vi "PicoScope6000GetRapidBlock.vi"(0 "error in":errorcluster, 7 "handle in":i16, 11 "Rapid Block Acquisition Settings":T1) -> (2 "Channel A Buffer":i16[][](array[numeric]), 3 "Channel B Buffer":i16[][](array[numeric]), 4 "error out":errorcluster, 6 "handle out":i16, 13 "Channel C Buffer":i16[][](array[numeric]), 14 "Channel D Buffer":i16[][](array[numeric]))   [LabVIEW 2009]
doc: "This VI gets a set of blocks captured using rapid block mode. It outputs two-dimensional arrays for each channel that contain data from all the requested captures."
uses:
  PS6000.dll
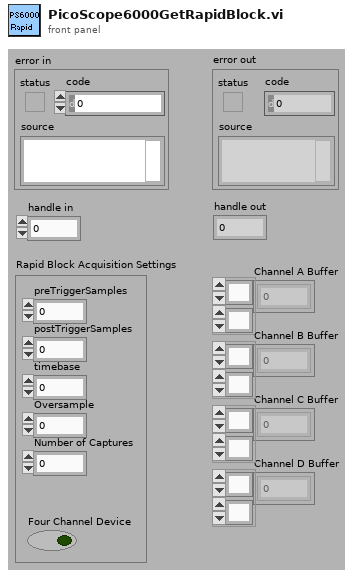
[diagram p1: front panel]
types:
  T1 = cluster{"preTriggerSamples":u32, "postTriggerSamples":u32, "timebase":u32, "Four Channel Device":bool, "Oversample":i16, "Number of Captures":u32}
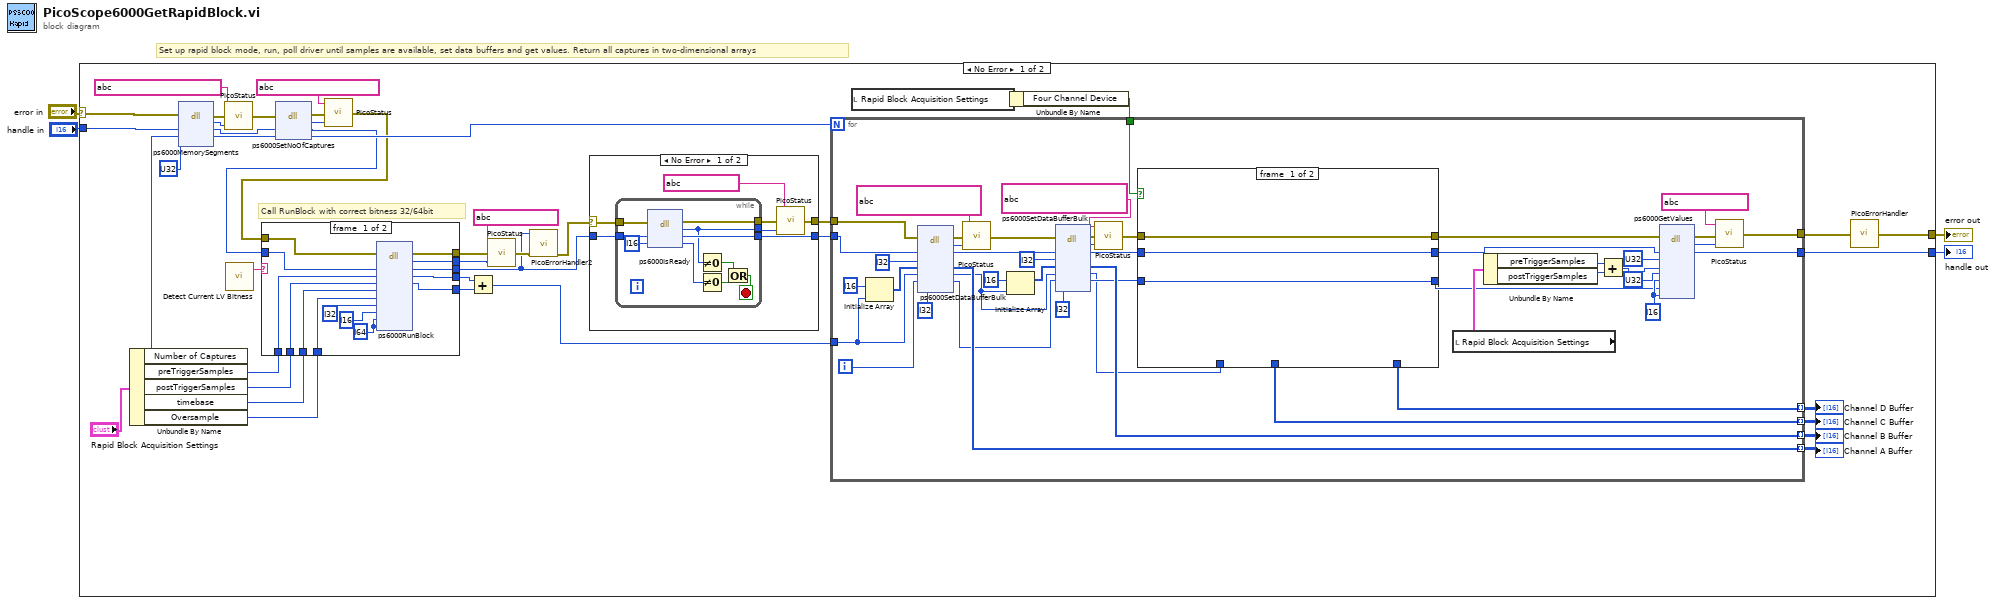
[diagram p0: block diagram]
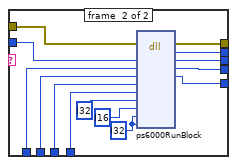
[diagram p2: hidden frame]
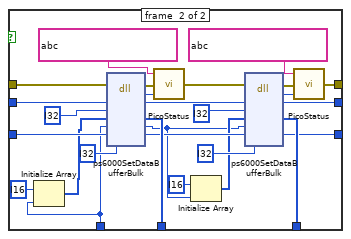
[diagram p3: hidden frame]
diagram:
  # "Set up rapid block mode, run, poll driver until samples are available, set data buffers and get values. Return all captures in two-dimensional arrays"
  n1 = case shown="No Error" "error in" {
    selector: "error in" -> [w42 w171]
    tunnel: [w21 w171] -> w3
    tunnel: "handle in" -> [w41 w170]
    tunnel: [w23 w170] -> w1
    frame #0 {
      # "Call RunBlock with correct bitness 32/64bit"
      n2 = Unbundle By Name("Rapid Block Acquisition Settings") -> ("Number of Captures"=w37:u32, "preTriggerSamples"=w9:u32, "postTriggerSamples"=w8:u32, "timebase"=w7:u32, "Oversample"=w6:i16)
      n3 = dll-call lib="PS6000.dll" fn="ps6000MemorySegments" ("ps3000.dll:_ps3000_open_unit@0")(error in=w42, "handle"=w41, "nSegments"=w37, "nMaxSamples"=u32 ?) -> (error out=w39:errorcluster, "PICO_STATUS"=w40:i32, "handle"=w34:i16, "nSegments"=w35:u32)  [unwired: 3 in, 1 out]
      n4 = call "PicoStatus.vi"("PICO STATUS"=w40, "error in"=w39, "source"=string ?) -> ("error out"=w33:errorcluster)
      n5 = call "Detect Current LV Bitness.vi"() -> ("bitness"=w16:string)  [unwired: 11 in]
      n6 = dll-call lib="PS6000.dll" fn="ps6000SetNoOfCaptures" ("ps3000.dll:_ps3000_open_unit@0")(error in=w33, "handle"=w34, "nCaptures"=w35) -> (error out=w31:errorcluster, "PICO_STATUS"=w32:i32, "handle"=w12:i16, "nCaptures"=w28:u32)  [unwired: 2 in, 1 out]
      n7 = call "PicoStatus.vi"("PICO STATUS"=w32, "error in"=w31, "source"=string ?) -> ("error out"=w13:errorcluster)
      n8 = case shown="\"32\", Default" w16 {
        tunnel: w7 -> [w60 w74]
        tunnel: w9 -> [w59 w73]
        tunnel: w8 -> [w58 w72]
        tunnel: [w57 w71] -> w20
        tunnel: [w56 w70] -> w19
        tunnel: w13 -> [w55 w69]
        tunnel: w12 -> [w54 w68]
        tunnel: w6 -> [w53 w67]
        tunnel: [w52 w66] -> w10
        tunnel: [w48 w62] -> w15
        tunnel: [w47 w61] -> w14
        frame #0 {
          w50 = i64 ? ("pParameter")
          n9 = dll-call lib="PS6000.dll" fn="ps6000RunBlock" ("ps3000.dll:_ps3000_open_unit@0")(error in=w55, "handle"=w54, "preTriggerSamples"=w59, "postTriggerSamples"=w58, "timebase"=w60, "oversample"=w53, "timeindisposed"=i32 ? ("pParameter"), "segmentIndex"=i16 ? ("pParameter"), "lpReady"=w50, "pParameter"=w50) -> (error out=w56:errorcluster, "PICO_STATUS"=w57:u32, "handle"=w52:i16, "preTriggerSamples"=w47:u32, "postTriggerSamples"=w48:u32)  [unwired: 8 in, 1 out]
        }
        frame #1 {
          w64 = i32 ? ("pParameter")
          n10 = dll-call lib="PS6000.dll" fn="ps6000RunBlock" ("ps3000.dll:_ps3000_open_unit@0")(error in=w69, "handle"=w68, "preTriggerSamples"=w73, "postTriggerSamples"=w72, "timebase"=w74, "oversample"=w67, "timeindisposed"=i32 ? ("pParameter"), "segmentIndex"=i16 ? ("pParameter"), "lpReady"=w64, "pParameter"=w64) -> (error out=w70:errorcluster, "PICO_STATUS"=w71:u32, "handle"=w66:i16, "preTriggerSamples"=w61:u32, "postTriggerSamples"=w62:u32)  [unwired: 8 in, 1 out]
        }
      }
      n11 = Add(x=w14, y=w15) -> (x+y=w5:u32)
      n12 = call "PicoStatus.vi"("PICO STATUS"=w20, "error in"=w19, "source"=string ?) -> ("error out"=w17:errorcluster)
      n13 = call "PicoErrorHandler2.vi"("error in (no error)"=w17, "handle In"=w10) -> ("error out"=w11:errorcluster)  [unwired: 9 in]
      n14 = case shown="No Error" w11 {
        selector: w11 -> [w155 w168]
        tunnel: w10 -> [w157 w169]
        tunnel: [w156 w169] -> w46
        tunnel: [w154 w168] -> w45
        frame #0 {
          n15 = while {
            tunnel: [w167] -> w156
            tunnel: w157 -> [w166]
            tunnel: [w161] -> w152
            tunnel: w155 -> [w160]
            tunnel: [w159] -> w153
            stop <- w165 stop-if-true
            n16 = dll-call lib="PS6000.dll" fn="ps6000IsReady" ("ps3000.dll:_ps3000_open_unit@0")(error in=w160, "handle"=w166, "ready"=i16 ?) -> (error out=w159:errorcluster, "status"=w161:i32, "handle"=w167:i16, "ready"=w162:i16)  [unwired: 2 in, 1 out]
            n17 = Not Equal To 0?(x=w161) -> (x != 0?=w163:bool)
            n18 = Not Equal To 0?(x=w162) -> (x != 0?=w164:bool)
            n19 = Or(x=w163, y=w164) -> (x .or. y?=w165:bool)
          }
          n20 = call "PicoStatus.vi"("PICO STATUS"=w152, "error in"=w153, "source"=string ?) -> ("error out"=w154:errorcluster)
        }
        frame #1 {
        }
      }
      n21 = local read "Rapid Block Acquisition Settings"() -> (w29:T1)
      n22 = Unbundle By Name(w29) -> ("Four Channel Device"=w43:bool)
      n23 = for {
        N: w28 -> [_]
        tunnel: w46 -> [w120]
        tunnel: w45 -> [w115]
        tunnel: w43 -> [w106]
        tunnel: [w109] -> w27 mode=indexing
        tunnel: [w108] -> w26 mode=indexing
        tunnel: [w82] -> w25 mode=indexing
        tunnel: [w104] -> w24 mode=indexing
        tunnel: w5 -> [w107]
        tunnel: [w91] -> w23
        tunnel: [w77] -> w22
        i -> [w105]
        w103 = i16 ? ("overflow")
        n24 = Initialize Array(i16 ? ("element"), w107) -> (w119:i16[])
        n25 = dll-call lib="PS6000.dll" fn="ps6000SetDataBufferBulk" ("ps3000.dll:_ps3000_open_unit@0")(error in=w115, "handle"=w120, "channel"=i32 ?, "buffer"=w119, "bufferLth"=w107, "waveform"=w105, "downSampleRatioMode"=i32 ?) -> (error out=w113:errorcluster, "PICO_STATUS"=w114:i32, "handle"=w87:i16, "buffer"=w104:i16[], "bufferLth"=w84:u32, "waveform"=w83:u32)  [unwired: 4 in, 1 out]
        n26 = call "PicoStatus.vi"("PICO STATUS"=w114, "error in"=w113, "source"=string ?) -> ("error out"=w88:errorcluster)
        n27 = Initialize Array(i16 ? ("element"), w84) -> (w85:i16[])
        n28 = dll-call lib="PS6000.dll" fn="ps6000SetDataBufferBulk" ("ps3000.dll:_ps3000_open_unit@0")(error in=w88, "handle"=w87, "channel"=i32 ?, "buffer"=w85, "bufferLth"=w84, "waveform"=w83, "downSampleRatioMode"=i32 ?) -> (error out=w90:errorcluster, "PICO_STATUS"=w89:i32, "handle"=w81:i16, "buffer"=w82:i16[], "bufferLth"=w75:u32, "waveform"=w80:u32)  [unwired: 4 in, 1 out]
        n29 = call "PicoStatus.vi"("PICO STATUS"=w89, "error in"=w90, "source"=string ?) -> ("error out"=w112:errorcluster)
        n30 = case shown="True" w106 {
          tunnel: w81 -> [w123 w142]
          tunnel: [w123 w136] -> w93
          tunnel: [_ w138] -> w109
          tunnel: [_ w145] -> w108
          tunnel: w112 -> [w122 w141]
          tunnel: [w122 w150] -> w94
          tunnel: w75 -> [_ w125]
          tunnel: w80 -> [w121 w144]
          tunnel: [w121 w137] -> w92
          frame #0 {
          }
          frame #1 {
            n31 = Initialize Array(i16 ? ("element"), w125) -> (w128:i16[])
            n32 = dll-call lib="PS6000.dll" fn="ps6000SetDataBufferBulk" ("ps3000.dll:_ps3000_open_unit@0")(error in=w141, "handle"=w142, "channel"=i32 ?, "buffer"=w128, "bufferLth"=w125, "waveform"=w144, "downSampleRatioMode"=i32 ?) -> (error out=w147:errorcluster, "PICO_STATUS"=w146:i32, "handle"=w135:i16, "buffer"=w145:i16[], "bufferLth"=w124:u32, "waveform"=w132:u32)  [unwired: 4 in, 1 out]
            n33 = call "PicoStatus.vi"("PICO STATUS"=w146, "error in"=w147, "source"=string ?) -> ("error out"=w134:errorcluster)
            n34 = Initialize Array(i16 ? ("element"), w124) -> (w126:i16[])
            n35 = dll-call lib="PS6000.dll" fn="ps6000SetDataBufferBulk" ("ps3000.dll:_ps3000_open_unit@0")(error in=w134, "handle"=w135, "channel"=i32 ?, "buffer"=w126, "bufferLth"=w124, "waveform"=w132, "downSampleRatioMode"=i32 ?) -> (error out=w140:errorcluster, "PICO_STATUS"=w139:i32, "handle"=w136:i16, "buffer"=w138:i16[], "waveform"=w137:u32)  [unwired: 5 in, 1 out]
            n36 = call "PicoStatus.vi"("PICO STATUS"=w139, "error in"=w140, "source"=string ?) -> ("error out"=w150:errorcluster)
          }
        }
        n37 = local read "Rapid Block Acquisition Settings"() -> (w99:T1)
        n38 = Unbundle By Name(w99) -> ("preTriggerSamples"=w101:u32, "postTriggerSamples"=w100:u32)
        n39 = Add(x=w101, y=w100) -> (x+y=w102:u32)
        n40 = dll-call lib="PS6000.dll" fn="ps6000GetValues" ("ps3000.dll:_ps3000_open_unit@0")(error in=w94, "handle"=w93, "startIndex"=u32 ?, "noOfSamples"=w102, "downSampleRatio"=u32 ?, "downSampleRatioMode"=w103, "segmentIndex"=w92, "overflow"=w103) -> (error out=w96:errorcluster, "PICO_STATUS"=w95:i32, "handle"=w91:i16)  [unwired: 8 in, 1 out]
        n41 = call "PicoStatus.vi"("PICO STATUS"=w95, "error in"=w96, "source"=string ?) -> ("error out"=w77:errorcluster)
      }
      "Channel D Buffer" <- w27
      "Channel C Buffer" <- w26
      "Channel B Buffer" <- w25
      "Channel A Buffer" <- w24
      n42 = call "PicoErrorHandler.vi"("error in"=w22) -> ("error out"=w21:errorcluster)
    }
    frame #1 {
    }
  }
  "error out" <- w3
  "handle out" <- w1
